vi "总氮流程质控自动启动.vi"(10 "总氮量程切换":enum32{"H", "L", "AUTO"}(ring)=enum."AUTO", 11 "参数":T1={"是否启用仪器"=FALSE, "CODMn"={"启动测量模式"={"测量模式"=enum."水样测量"}, "确定按钮"=TRUE}, "启动模块"={"氨氮"=FALSE, "总磷"=FALSE, "总氮"=FALSE, "COD"=FALSE}, "常规启动"=FALSE, "直接启动"=FALSE}) -> ()   [LabVIEW 2016, in "质控单元.lvlib"]
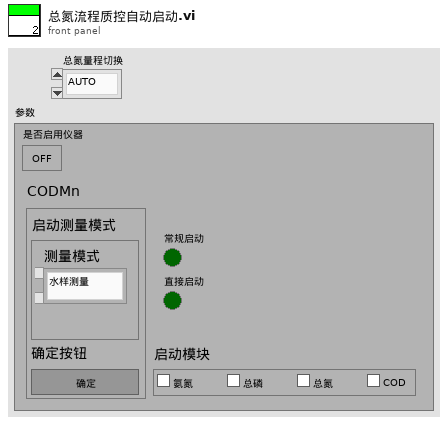
[diagram p1: front panel]
types:
  T1 = cluster{"是否启用仪器":bool, "CODMn":cluster{"启动测量模式":cluster{"测量模式":enum16{"水样测量", "标样核查", "加标回收", "平行样", "校零", "校标"}}, "确定按钮":bool}, "启动模块":cluster{"氨氮":bool, "总磷":bool, "总氮":bool, "COD":bool}, "常规启动":bool, "直接启动":bool}
  T2 = cluster{"R0":i16, "R1":i16, "R2":i16, "R3":i16, "R4":i16, "R5":i16, "R6":i16, "R7":i16, "R8":i16, "R9":i16, "R10":i16, "R11":i16, "R12":i16, "R13":i16, "R14":i16, "R15":i16, "R16":i16, "R17":i16, "R18":i16, "R19":i16, "R20":i16, "R21":i16, "R22":i16, "R23":i16, "R24":i16, "R25":i16, "R26":i16, "R27":i16, "R28":i16, "R29":i16, "R30":i16, "R31":i16, "R32":i16, "R33":i16, "R34":i16, "R35":i16, "R36":i16, "R37":i16, "R38":i16, "R39":i16, "R40":i16, "R41":i16, "R42":i16, "R43":i16, "R44":i16, "R45":i16, "R46":i16, "R47":i16, "R48":i16, "R49":i16, "R50":i16, "R51":i16, "R52":i16, "R53":i16, "R54":i16, "R55":i16, "R56":i16}
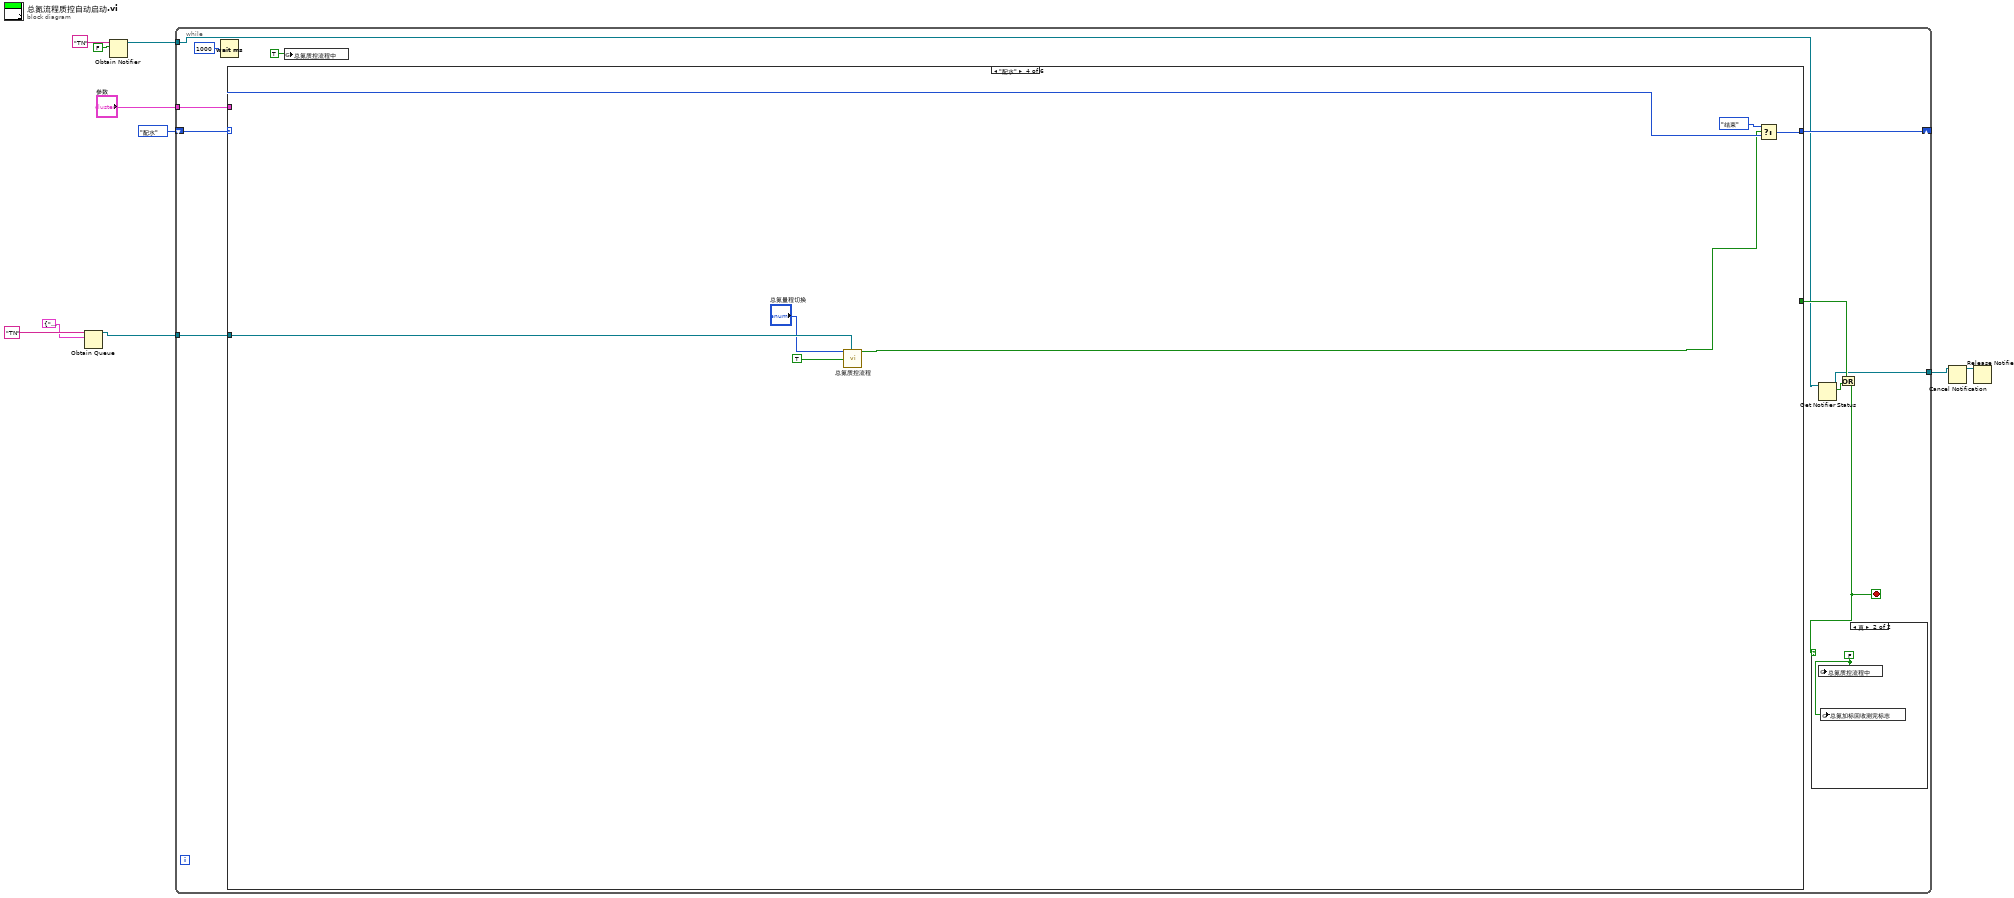
[diagram p0: block diagram]
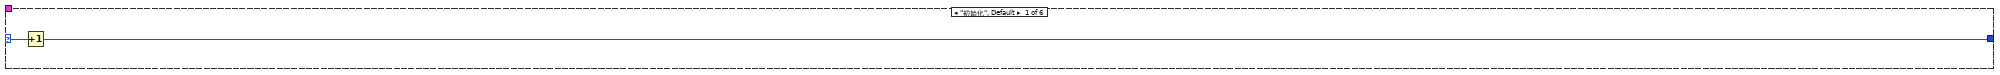
[diagram p3: hidden frame]
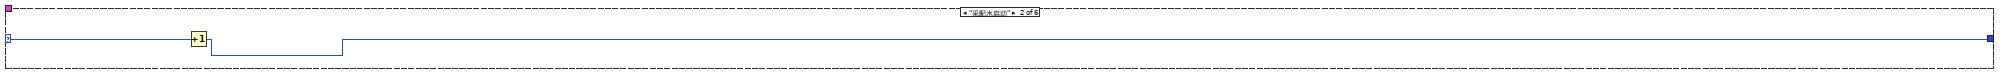
[diagram p4: hidden frame]
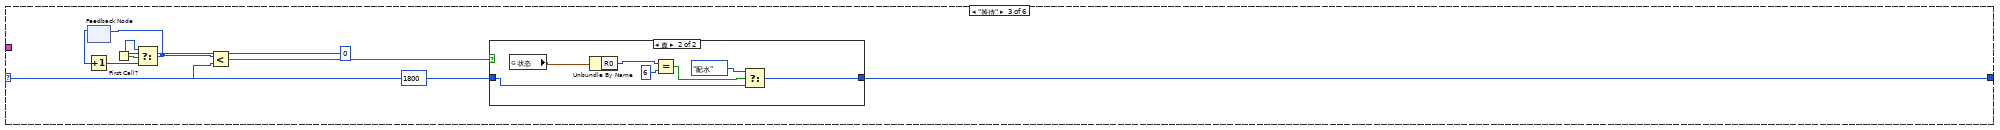
[diagram p5: hidden frame]
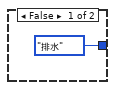
[diagram p6: hidden frame]
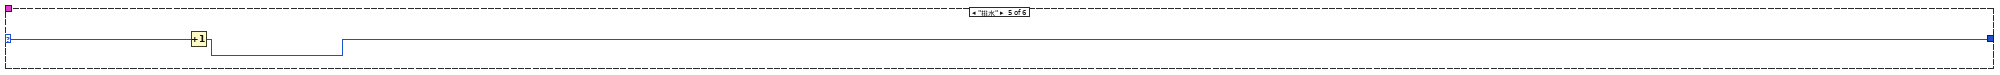
[diagram p7: hidden frame]
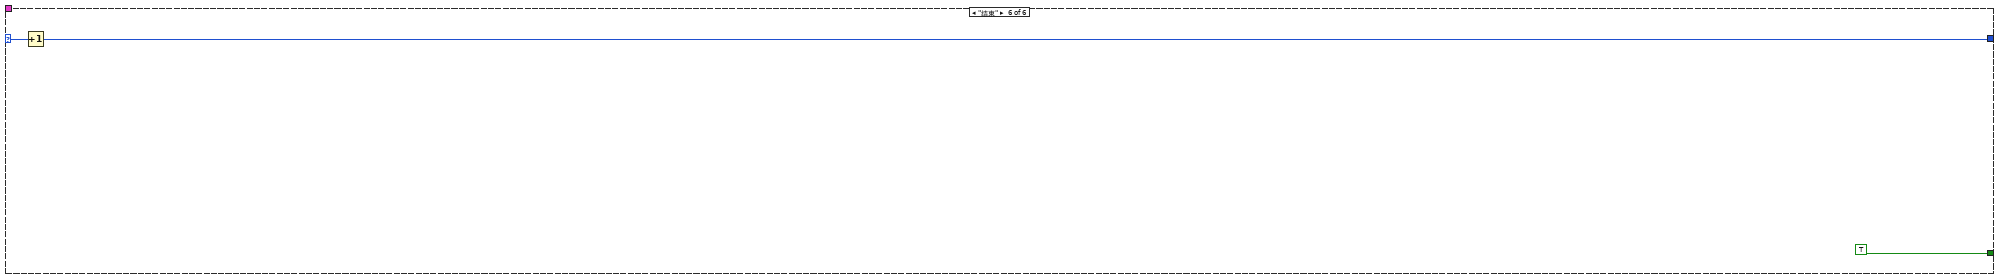
[diagram p8: hidden frame]
diagram:
  n1 = Obtain Queue(name (unnamed)="TN" ("名称（未命名）"), element data type=cluster{"命令":string, "data":variant} {"命令"="", "data"=variant}) -> (queue out=w1:refnum<queue>)  [unwired: 3 in, 2 out]
  n2 = Obtain Notifier(name (unnamed)="TN" ("名称（未命名）"), notification data type=FALSE) -> (notifier out=w6:refnum<notifier>)  [unwired: 2 in, 2 out]
  n3 = while {
    shift-right: [w20] -> _
    shift-left: enum16{"初始化", "采配水启动", "等待", "配水", "排水", "结束"}."配水" ("枚举") -> [w21]
    tunnel: "参数" -> [w18]
    tunnel: w1 -> [w17]
    tunnel: w6 -> [w15]
    tunnel: [w13] -> w4
    stop <- w11 stop-if-true
    n4 = Wait (ms)(milliseconds to wait=u32 1000 ("等待时间（毫秒）")) -> ()  [unwired: 1 out]
    n5 = case shown="\"配水\"" w21 {
      selector: w21 -> [w24 w26 w33 w49 w52 w55]
      tunnel: [w23 w25 w32 w48 w51 w54] -> w20
      tunnel: [_ _ _ _ _ TRUE] -> w16
      tunnel: w18 -> [_ _ _ _ _ _]
      tunnel: w17 -> [_ _ _ w46 _ _]
      frame "初始化", Default {
        n6 = Increment(x=w24) -> (x+1=w23:enum16{"初始化", "采配水启动", "等待", "配水", "排水", "结束"})
      }
      frame "采配水启动" {
        n7 = Increment(x=w26) -> (x+1=w25:enum16{"初始化", "采配水启动", "等待", "配水", "排水", "结束"})
      }
      frame "等待" {
        n8 = feedback #1() -> (w29:i32)  [unwired: 1 in]
        n9 = Increment(x=w29) -> (x+1=w28:i32)
        n10 = First Call?() -> (First Call?: T/F=w30:bool)
        n11 = Select(t=0, s=w30, f=w28) -> (s? t:f=w27:i32)
        n12 = feedback-in #1(w27) -> ()
        n13 = Less?(x=w27, y=1800) -> (x < y?=w34:bool)
        n14 = case shown="真" w34 {
          tunnel: w33 -> [_ w39]
          tunnel: [enum16{"初始化", "采配水启动", "等待", "配水", "排水", "结束"}."排水" ("枚举") w38] -> w32
          frame False {
          }
          frame True {
            n15 = global read "与采配水交互全局.vi" "状态"() -> (w37:T2)
            n16 = Unbundle By Name(w37) -> ("R0"=w43:i16)
            n17 = Equal?(x=w43, y=i16 6) -> (x = y?=w41:bool)
            n18 = Select(t=enum16{"初始化", "采配水启动", "等待", "配水", "排水", "结束"}."配水" ("枚举"), s=w41, f=w39) -> (s? t:f=w38:enum16{"初始化", "采配水启动", "等待", "配水", "排水", "结束"})
          }
        }
      }
      frame "配水" {
        n19 = call "总氮质控流程.vi"("队列输入TN"=w46, "总氮"=TRUE ("氨氮"), "总氮量程切换"="总氮量程切换") -> ("布尔"=w47:bool)  [unwired: 7 in]
        n20 = Select(t=enum16{"初始化", "采配水启动", "等待", "配水", "排水", "结束"}."结束" ("枚举"), s=w47, f=w49) -> (s? t:f=w48:enum16{"初始化", "采配水启动", "等待", "配水", "排水", "结束"})
      }
      frame "排水" {
        n21 = Increment(x=w52) -> (x+1=w51:enum16{"初始化", "采配水启动", "等待", "配水", "排水", "结束"})
      }
      frame "结束" {
        n22 = Increment(x=w55) -> (x+1=w54:enum16{"初始化", "采配水启动", "等待", "配水", "排水", "结束"})
      }
    }
    n23 = global write "质控测完标志全局 1.vi" "总氮质控流程中"(TRUE ("氨氮质控流程中")) -> ()
    n24 = Get Notifier Status(notifier=w15) -> (notifier out=w13:refnum<notifier>, current notification=w14:bool)  [unwired: 1 in, 3 out]
    n25 = Or(x=w16, y=w14) -> (x .or. y?=w11:bool)
    n26 = case shown="真" w11 {
      frame False {
      }
      frame True {
        w22 = FALSE ("氨氮质控流程中")
        n27 = global write "质控测完标志全局 1.vi" "总氮质控流程中"(w22) -> ()
        n28 = global write "质控测完标志全局 1.vi" "总氮加标回收测完标志"(w22) -> ()
      }
    }
  }
  n29 = Cancel Notification(0:w4) -> (8:w5:refnum<notifier>)  [unwired: 1 in, 2 out]
  n30 = Release Notifier(notifier=w5) -> ()  [unwired: 2 in, 3 out]
